vi "Notify Completion.vi"(8 "error in (no error)":errorcluster, 10 "Async Message":refnum<class "Async Message.lvclass">, 11 "Async Methods Actor in":refnum<class "Async Methods Actor.lvclass">) -> (0 "error out":errorcluster, 3 "Async Methods Actor out":refnum<class "Async Methods Actor.lvclass">)   [LabVIEW 2021, in "Async Methods Actor.lvlib" / "Async Methods Actor.lvclass"]
uses:
  Async Methods Actor.lvclass
  Async Methods Actor Messages/Async Message/Async Message.lvclass
  C:/Program Files/National Instruments/LabVIEW 2021/vi.lib/ActorFramework/Message/Message.lvclass
  Async Methods Actor Messages/Completion Notification Msg/Completion Notification Data.ctl
  Async Methods Actor.lvclass/Async Methods Actor.ctl
  Async Methods Actor Messages/Async Message/Async Message.lvclass/Async Message.ctl
  Async Methods Actor Messages/Completion Notification Msg/Completion Notification Msg.lvclass/Completion Notification Msg.ctl
  <vilib>/ActorFramework/Message Enqueuer/Message Enqueuer.lvclass/Message Enqueuer.ctl
  Async Methods Actor Messages/Async Message/Read FQN.vi
  Async Methods Actor Messages/Async Message/Read Caller Enqueuer.vi
  Async Methods Actor Messages/Async Message/Read Completion Notification Msg.vi
  <vilib>/ActorFramework/Message Enqueuer/Enqueue.vi
  Get VI FQN.vi
  Async Methods Actor Messages/Completion Notification Msg/Completion Notification Msg.lvclass
  <vilib>/Utility/LVClass/Get LV Class Path.vi
  <vilib>/ActorFramework/Message Priority Queue/Priority Enqueue.vi
  <vilib>/ActorFramework/Message Enqueuer/Message Enqueuer.lvclass
  <vilib>/ActorFramework/Message/Message.lvclass
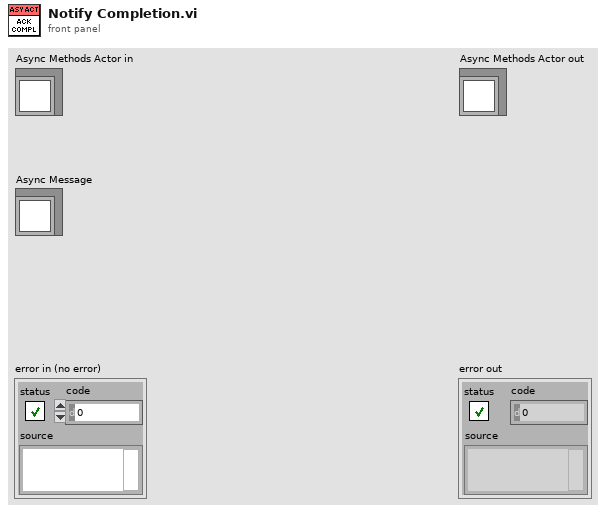
[diagram p1: front panel]
types:
  T1 = typedef "Async Methods Actor.lvlib/Completion Notification Msg.lvclass/Completion Notification Data.ctl" = cluster{"Async Message":refnum<class "Async Message.lvclass">, "Current Execution Count":u32}
  T2 = typedef "Async Methods Actor.lvlib/Async Methods Actor.lvclass/Async Message Execution Status Map.ctl" = map{string, T3}
  T3 = typedef "Async Methods Actor.lvlib/Async Methods Actor.lvclass/Async Message Execution Status.ctl" = cluster{"C&C Clones Running":u32, "C&F Clones Launched":u32}
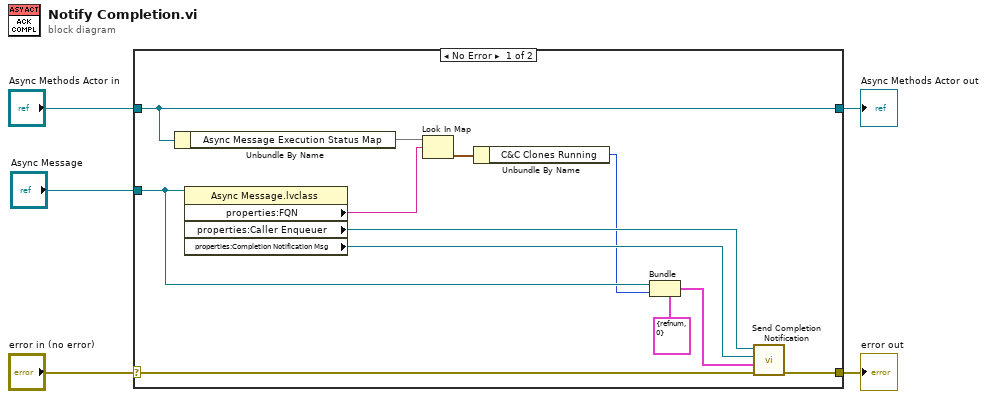
[diagram p0: block diagram]
diagram:
  n1 = case shown="No Error" "error in (no error)" {
    selector: "error in (no error)" -> [w9 w19]
    tunnel: [w8 w19] -> w4
    tunnel: [w17 w18] -> w2
    tunnel: "Async Methods Actor in" -> [w17 w18]
    tunnel: "Async Message" -> [w13 _]
    frame No Error {
      n2 = Unbundle By Name(w17) -> ("Async Message Execution Status Map"=w16:T2)
      n3 = property class="Async Message.lvclass"(reference=w13) -> ("properties:FQN"=w12:string, "properties:Caller Enqueuer"=w10:refnum<class "Message Enqueuer.lvclass">, "properties:Completion Notification Msg"=w7:refnum<class "Completion Notification Msg.lvclass">)  [unwired: 1 in, 2 out]
      n4 = Look In Map(map=w16, key=w12) -> (value=w15:T3)  [unwired: 1 in, 1 out]
      n5 = Unbundle By Name(w15) -> ("C&C Clones Running"=w6:u32)
      n6 = Bundle(cluster=T1 {"Async Message"=refnum, "Current Execution Count"=0} ("Completion Ack Data"), "Async Message"=w13, "Current Execution Count"=w6) -> (w11:T1)
      n7 = call "Send Completion Notification.vi"("error in (no error)"=w9, "Completion Notification Data"=w11, "Message Type"=w7, "Message Enqueuer"=w10) -> ("error out"=w8:errorcluster)  [unwired: 6 in, 1 out]
    }
    frame Error {
    }
  }
  "error out" <- w4
  "Async Methods Actor out" <- w2
